vi "Atto DRY Interface get Cryostat In Valve.vi"(8 "error in (no error)":errorcluster, 11 "valveStatus":i32) -> (0 "error out":errorcluster, 2 "function return":i32, 3 "valveStatus out":i32)   [LabVIEW 2016, in "attoDRYLib.lvlib"]
doc: "int32_t __cdecl AttoDRY_Interface_getCryostatInValve(int *valveStatus);"
uses:
  <userlib>/attoDRYLib/attoDRYLib.lvlib
  <userlib>/attoDRYLib/attoDRYLib.dll
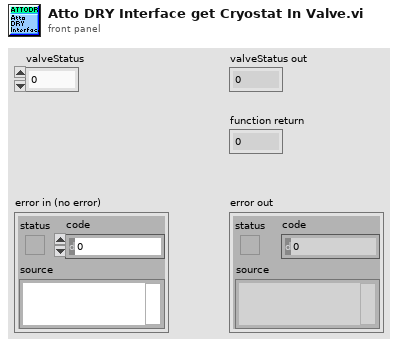
[diagram p1: front panel]
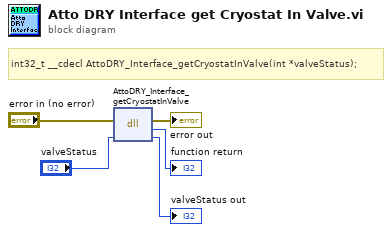
[diagram p0: block diagram]
diagram:
  # "int32_t __cdecl AttoDRY_Interface_getCryostatInValve(int *valveStatus);"
  n1 = dll-call lib="C:/Program Files (x86)/National Instruments/LabVIEW 2016/user.lib/attoDRYLib/attoDRYLib.*" fn="AttoDRY_Interface_getCryostatInValve"(error in="error in (no error)", "valveStatus"="valveStatus") -> (error out=→"error out":errorcluster, →"function return":i32, "valveStatus"=→"valveStatus out":i32)  [unwired: 2 in, 1 out]
